vi "transceive.vi"() -> ()   [LabVIEW 2020]
uses:
  <vilib>/measure/matone.llb/Extract Single Tone Information 1 Chan (CDB).vi
  <vilib>/measure/maspectr.llb/FFT Power Spectrum and PSD for 1 Chan (CDB).vi
  <vilib>/measure/NI_MABase.lvlib
  <vilib>/measure/NI_MAPro.lvlib
panel:
  in  "stop":bool
  out "Package Directory":path
  out "Transmit Stop?":bool
  out "Terminal Output":string
  in  "FMC Parameters":T1={"IP"="169.254.92.202", "Port"=22, "Username"="analog", "Password"="analog", "Tx rfPort"="A", "Tx Frequency"=2400, "Sample Rate"=30.72, "Tx Bandwidth"=18, "Tx Attenuation"=0, "Cyclic?"=TRUE, "Rx rfPort"="A", "Rx Frequency"=2400, "Rx Bandwidth"=18, "Num of Samples"=16384, "RxA Att"=0.0, "Rx Gain"=0.0}
  in  "?":enum32{"Transmitted Data", "Rx Time", "Rx Freq"}(tab)
  out "Transmitted Waveform":waveform(dbl)[](graph)
  out "Received Waveform":dbl[][](graph)
  out "PSD":cluster{"f0":dbl, "df":dbl, "magnitude":dbl[]}(graph)={"f0"=-0.5, "df"=0.0009765625, "magnitude"=[-2.1664662387993214, -11.03031844193236, -16.21298370209194, -4.2080616825271475, -1.8741588804049676, 1.1653000889131602, -1.8891898884953007, -2.864952815094211, -21.184075663903045, -6.459011634389907, -9.425575045654224, -3.690679662683627, -1.9755112973017053, -12.88760998423885, -7.142795197511936, -5.749654993033601, -4.232121719401448, -6.5853324526702135, -16.72201576955071, -9.904618860083986, -3.7536909694395684, -11.12706914338175, -2.8284209492202423, -4.69775383894684, -1.81721905978906, 2.6751922066707197, -6.228922467094204, -8.725900475207114, -3.2266453224266387, 0.7951367070723341, 3.18791480156189, 1.146568401648937, -15.284613684557055, -7.029959998724905, -9.547309724544128, -9.641529484569087, -4.012009186143547, -2.007072588608481, -2.7914766687377783, -2.6237078006362573, -4.309788836088561, -18.475581742500292, -4.870258369106881, -2.025766794368759, -4.321152799180626, -7.919073671305048, -9.634049825771205, -9.066188593143584, -0.5305564612559043, -0.31734285019072245, -2.899678030076754, -4.930580506434592, -5.89966356805042, -7.472329086898343, -3.2393794433644625, 2.8054749156287695, 1.101964532151964, -4.615302488116255, -6.950562817482371, -6.012731538910917, -6.136893822759926, -4.6471679348476655, -1.2244038951072234, -4.415810566038147, -10.277196994849163, -6.747298439500046, -9.345274520940713, -24.63822602993131, -9.626589129035054, -12.030032194659979, -8.307672166916715, -4.925425049785537, -6.599824942748922, -14.48643716405336, -4.097115992439623, -4.577980789198419, -7.890347310753404, -19.88220101638118, -4.378072425832935, -5.46719551585171, -5.179404332980243, -1.0377130577596902, -10.067538970313956, -3.9345824246573313, -7.348762210999691, -4.4813140018042255, -13.322269126358782, -18.614476297439715, -11.901757888638036, -15.494707432373744, -2.5504818043536654, -0.39477467835974145, -2.304623583891613, -1.7011053039774162, -1.0588041474234957, -5.7947060018517025, -6.930737241367428, -11.138280621615529, -3.142790539526048, -4.1349241709963085, -6.493611114179859, -13.668598830892726, -6.06473945193608, -4.573451548903187, -12.681769905622991, -10.520049431046665, -11.196572091425558, -3.080583619040455, -1.1668660568295595, -10.149043360414288, -14.050701122230615, -23.29131249709334, -25.61066622144638, -7.28124149909767, -4.729883842869232, -5.731993156566849, -9.19277681711874, -16.35268142406711, -18.644837970125387, -9.055595050639003, -5.065337383658032, -5.737763649573261, -8.955349256338103, -8.614404932103014, -18.012974581333005, -10.62396244470849, -13.554883384566025, -11.053708375035576, -13.814110268725772, -10.341204454518444, -11.601018866430993, -9.480774966741487, -14.773641827392439, -11.639321854216638, -5.276785459852072, -3.389349753355969, -9.62066285902237, -13.704466876991075, -15.356678941850866, -11.090197312926346, -15.765625988870731, -19.504916189187135, -11.722808010214179, -7.598506986517483, -4.505296743673027, -5.822883424781482, -16.09011596093657, -14.043949050340707, -16.089051948303435, -9.487296265628675, -15.128223317596767, -10.018626031429827, -9.267900156035067, -8.380021959177236, -13.476338432933685, -7.208337471083226, -13.354661158796306, -9.04978003921784, -16.012521467074837, -11.961586037421164, -10.924513690003696, -15.265653652735791, -21.78119293221372, -23.444167957273756, -18.99901373597104, -9.661919978212918, -8.769352364462925, -9.287529637864772, -11.285381835174613, -11.978298753836219, -14.12055103294531, -19.629285771576967, -14.884787585567448, -20.815518177082293, -14.164324358055287, -8.780900988880223, -11.738326415102133, -16.152955231194802, -17.32671574436486, -14.838120659422156, -19.05492324460187, -20.95423425206988, -17.5564628136197, -11.578639978063084, -14.486427948155738, -26.34134938136794, -13.688104874335611, -8.57434558212727, -10.449000554689265, -15.905851233765231, -27.66525811513363, -16.0113299515765, -20.040788269819906, -14.555987823168017, -9.646150758194366, -11.27934438013196, -14.566967642712562, -15.132750471219198, -21.40247412832394, -18.07051340158898, -25.17678076571924, -18.78255043567815, -16.45857022203186, -17.443314784160325, -22.145987897198967, -25.718710724338898, -24.544041374309064, -25.384442312132464, -55.16060392584162, -22.108378284322097, -17.760182487108363, -16.197006612175016, -15.734079533899587, -20.285641706516017, -20.491143754075583, -14.564418592526122, -15.741471379702684, -18.511482132849927, -17.809104927296914, -15.124735483684024, -17.619988546039153, -17.85107813457279, -16.929723198620195, -20.948588507870348, -24.0715805700717, -18.118791892009778, -14.262411465607217, -12.299255622076606, -17.79348030858842, -27.607132100714807, -31.523131614059388, -20.31173109515901, -18.375492924569116, -29.91411408852937, -21.431199855002262, -35.5719476973811, -31.028910314184294, -17.602948806381388, -11.422758376296168, -15.796797787853741, -25.905898919356236, -23.309551487188443, -23.56295813940394, -24.9018395326393, -14.308676256089425, -12.644084832963776, -13.954709280494242, -11.568644948187757, -14.614471395213165, -16.83755663945805, -19.316516942378257, -17.622380146368744, -25.38633973795314, -21.367209508959995, -16.67367263138378, -19.022940164088457, -23.968867457596076, -18.111523749501185, -20.158096530028146, -37.615159078310356, -29.73443523402027, -21.712570154675362, -17.774184712470547, -15.506439974547515, -18.562298886616663, -22.88136665916835, -30.92169802339641, -21.059024146049175, -25.552942745021774, -21.776350752149266, -17.530732077159755, -31.369212824553937, -25.105693408622894, -24.372264823560283, -33.91496361346293, -44.72514042785862, -31.04986529591511, -21.39757719194284, -19.991438630226362, -26.34113093177384, -25.84372064517313, -41.748828296403246, -50.48308638460183, -25.421782746303705, -21.935572022862427, -25.368831172623732, -23.90029815548064, -27.074842703290795, -26.158836731751116, -45.411822297777576, -33.86289987595039, -27.872429800965705, -22.446348719121257, -20.502898835792827, -22.345505115510175, -26.643199128152837, -27.716256183557814, -30.43562805608401, -31.91587304586699, -31.2189770891335, -22.8004431029588, -20.463273944792533, -19.37577279279427, -23.775090890229187, -25.782381831922923, -19.676979008748468, -16.937682367459466, -17.5363763173867, -16.420024272236063, -25.164465188456727, -33.73845657221404, -20.065432217663293, -17.520338123580647, -18.750970185274095, -23.902417125492512, -17.07842144571978, -20.652237374407857, -18.34940376696168, -16.46552380797614, -20.25463508958933, -26.79551422437222, -35.67225613415172, -31.047698747465926, -21.268584472975057, -20.646197880367275, -23.518125515414525, -21.652181944937094, -23.208992746835015, -37.70332329061807, -28.49033175719009, -28.225438942675968, -38.79368719898007, -32.82324235723701, -24.214741268728226, -20.138091046784115, -24.47583216925584, -24.65584570012096, -21.53710617559499, -17.789621621098938, -23.016655485388668, -21.33131937730605, -18.96241963232589, -23.306139096559974, -31.77524183835225, -24.193632784059048, -40.79923068575879, -26.673785570437524, -19.91419651268278, -16.38621957158681, -25.037513134504504, -21.441693933714596, -17.271299896472755, -17.966366237189767, -22.947203587037187, -26.841391787104, -25.131401318506317, -17.174143861917088, -19.48010113279951, -15.986811775906064, -16.423921471328864, -21.19474324485939, -24.998695119051902, -22.54368429728293, -34.599609048332674, -26.642769012904175, -48.90868728146549, -26.424252509374067, -23.09570601456403, -21.44586205990473, -22.631979077558935, -22.630462483605292, -18.558161355724486, -21.21070987996529, -24.809823688147283, -28.111643763530555, -19.430787150252662, -18.934036484398895, -24.313645081015203, -24.052224792946827, -21.337203729576096, -26.310760265974885, -22.265681871887644, -18.12636200878271, -27.04230841618223, -26.78834309227041, -24.489069312961078, -18.71467432413909, -18.000186601341582, -21.258402666356005, -20.09803225228808, -20.166171669936954, -21.910662474230264, -27.805008936103718, -30.295775919638544, -20.355530298871475, -20.549721696850245, -19.177016446993573, -26.180585716564796, -31.99990225622599, -20.495928901318834, -19.893554597731963, -18.704938641767647, -16.266614210124846, -17.448229497012967, -21.23963887047376, -18.537721244758988, -22.59856844148533, -26.275140775135817, -23.8173694717668, -23.823056936129458, -24.637271758212908, -25.128701733314553, -20.061986995540472, -23.119809032129123, -28.36903214359627, -18.956044468969168, -18.702942936200742, -21.472616084356083, -19.327919866021922, -17.959722951763457, -18.591527190818006, -16.95060905889876, -19.32712734745809, -20.427199346264523, -31.226680872777273, -19.837382407924874, -22.60017932903269, -17.052777182725478, -20.40946447735477, -22.068669070393724, -20.81515564316504, -19.577957010052938, -20.099322802621508, -29.548811081650825, -26.12769052797335, -21.553209730395206, -19.13107867141223, -24.260238389039458, -27.286618589764757, -33.55279172848271, -21.272869637317534, -19.784506028159107, -26.78020113379997, -21.69964604589776, -24.629693542604922, -24.654456286565768, -15.229511185702185, -16.569856591164672, -25.727420831633523, -18.439246797446323, -15.41270238647343, -17.64852983558219, -27.525394034322925, -25.86016491040037, -17.034285316493328, -17.216011266586317, -17.77965679548461, -20.652685555422117, -25.11634227732326, -16.27916658908456, -19.904867479703867, -26.431609635922726, -25.400319119572327, -23.56382312081276, -21.874088081526608, -20.444656159001873, -36.40291084543626, -24.113336954401966, -24.9090995163475, -26.811296324942685, -18.85628812055225, -19.92832140194353, -17.719053554863546, -14.28207004215883, -17.01207225133356, -21.95767571091194, -16.83321472682335, -21.318257655642107, -21.987004143790692, -20.85570518163312, -22.09894380747681, -32.55333332110235, -29.72934345817011, -19.516577957830926, -17.287725402033377, -19.426934321453327, -21.876145018073018, -19.838378404678384, -21.294753350895476, -19.61650661591934, -23.735219067619013, -29.79064998014501, -30.65154385931423, -27.296316587055323, -22.463811070536956, -30.029030950678003, -23.723839332019715, -22.619765169322648, -21.87602943201536, -23.979099873473245, -26.33209423472927, -25.28676545037344, -24.513447334225354, -22.613416380850417, -28.445775896897572, -25.371972493999166, -26.95410699887337, -20.15755356935991, -29.342659520737925, -23.117020242869415, -22.600770165956984, -16.453300326319948, -12.132638160056581, -17.688216798310844, -20.33929698675172, -21.29991624897785, -22.229537539795302, -19.096565490704737, -28.140881490251157, -24.5329200204889, -24.27097199644253, -25.230287338715787, -23.43131783256496, -23.685264582837465, -25.877652372642412, -21.466251609993957, -19.76707428321712, -20.327234067749636, -23.16049957461841, -35.334331646673085, -26.20291010968397, -22.48453488096971, -22.521502075182678, -31.36991218027869, -29.541918177609592, -27.017269566287077, -24.165269959775163, -23.285450551161823, -31.1267069312302, -30.101399414709064, -21.41837897037453, -24.58127894254097, -33.675712305331146, -21.683603250949346, -23.46814135803816, -22.272480268297727, -20.303160142138484, -14.79328097819032, -17.54276386963902, -27.578074364075917, -27.188085587652218, -40.81262516669441, -27.1459170953992, -21.75914061223462, -18.91717204529973, -18.273575702330835, -22.64422421590675, -33.87762446569896, -22.226379927385153, -26.73584670700638, -24.67387294131232, -22.4854748232693, -36.31842033155398, -30.32832906473766, -27.623873893988407, -23.706361800320103, -39.28294513403284, -25.16384481375086, -29.14490096855095, -27.276793474720826, -30.22387754994218, -33.745621995360914, -21.13080065751321, -24.57667162525871, -21.40716783191923, -18.853149245032274, -20.87286216504811, -21.089605536097324, -21.433298698688983, -20.017338437952464, -22.091483642076778, -25.528526333253232, -20.9065418192947, -22.109035778048014, -40.61595229692652, -28.819683321057216, -28.16363103438912, -24.279230626850943, -18.06309619127601, -17.410855486281854, -29.253796833041918, -15.404729999237691, -25.143861834805232, -21.028188951021782, -23.59218835305257, -21.578422888284152, -25.68972331648026, -26.019146275513222, -18.029172276285372, -18.48357007669874, -17.659913594769137, -48.2437854268398, -18.302838627462748, -17.299244558802382, -18.627231694186637, -28.351797601823048, -21.655347673997255, -20.591819326458985, -29.42489293970261, -23.852565866915917, -36.15777214928648, -22.207740016509767, -20.296014432154223, -20.246050654007814, -26.856018528183263, -21.86136938534775, -19.244680908410075, -21.51739303579617, -20.056241624973538, -16.7222646629974, -18.859442838455404, -25.83383908787424, -23.305221121213794, -21.304054835291485, -25.820493558938878, -28.414975784284184, -27.767917030563783, -25.11334885337878, -22.792698450445776, -18.87117543186417, -20.73147740979615, -32.045486371077104, -25.098310761925866, -31.20757636259459, -21.387330527574377, -16.321479923262135, -16.58896228553176, -21.980872690771683, -42.02788785685936, -30.0006515278838, -18.757620854775755, -16.132462274618096, -23.637414124897695, -27.090364473222294, -21.86531457900997, -17.77321919544772, -16.949862714570273, -15.238539467356684, -15.730773682368644, -16.268405755729283, -17.328384424079417, -21.12891909300498, -20.194319845541898, -22.990301321132684, -27.632872106625342, -29.815486020850347, -53.437609513552296, -25.099883348901106, -28.050249905227513, -25.238353941682053, -18.920387452326143, -17.793562875056107, -18.05827559162568, -17.892584293097112, -23.626797056568552, -21.068850797989004, -19.37995435619343, -17.968181539408256, -15.534487272520627, -17.859497797480593, -22.742065600500155, -29.68362094699843, -24.635890295626982, -24.95482198228014, -24.38034414388111, -23.142504921877823, -18.86511676205624, -20.714811588589768, -24.28716238162186, -22.581457510652733, -28.731877346888396, -19.648954736106063, -24.61884036783917, -27.656612668890475, -19.40140716472233, -19.014493078107378, -29.674178521738995, -21.8969155384475, -19.99872387050329, -20.113178624244163, -21.9286770705693, -22.17623857618413, -24.910673474305725, -32.006128676967755, -23.41505068127347, -23.712189683586185, -29.899969415091476, -27.48158039751953, -27.706718959196195, -22.660148705331295, -19.40529056820971, -24.003963358719954, -28.86174279270587, -25.39456144991061, -28.023212416632308, -27.397584321546702, -28.638365635705302, -26.701711021434992, -37.32014723158207, -32.91599593470649, -33.21925099937459, -31.30991033598654, -31.2280941526455, -20.433366479115286, -19.87291267817699, -21.420416021206407, -17.33516761884006, -22.71233508900824, -24.419666766742655, -24.497763077045576, -24.5490781764792, -26.39950198033429, -24.715884025792644, -23.470016378188568, -21.382443036760783, -22.079530067255796, -18.561108520016898, -25.229058260292426, -24.802846865135237, -27.747385291793186, -27.20581202830468, -27.037703106072904, -19.47500379320967, -24.933467097925423, -21.915665157071697, -27.722597667704694, -20.20533713851103, -18.335532254847557, -20.205255402457034, -29.50280452603961, -25.68574081682002, -15.534415835980404, -13.405087901322457, -17.966232093133865, -26.798692490445877, -21.361673217922288, -15.429928071785666, -16.617493060665776, -27.080951843330816, -35.55964480499562, -26.547786417485064, -30.874533847630143, -23.306145626477832, -21.528398012495234, -31.90664483731751, -39.413438510354595, -19.3194963884024, -25.98808765766458, -26.606742660761906, -20.153792841684147, -19.613736231150096, -18.250265059418325, -27.097889502508735, -25.457471054870595, -28.02615784823974, -20.712914859368574, -23.062885911033568, -27.647652753943493, -21.757064606943942, -20.515510787449482, -21.148972569068505, -17.163549389658655, -14.128322318033199, -14.708517110823587, -21.13233507351331, -20.99462533980155, -11.033770144491386, -9.51961262575132, -19.740675685913384, -21.15896715801221, -18.272470374521454, -33.23019811130402, -20.817362450813217, -30.02135754202454, -19.3676160404167, -18.933303658417763, -21.889997993019634, -25.79689099190281, -25.65701279491698, -20.447890468062575, -17.507290471317308, -13.016197741038438, -11.67217989493539, -20.96905894781075, -15.26695904037564, -11.4928076833581, -12.775856238826167, -19.148804977158974, -26.141184946414917, -14.794321978537665, -14.630894652485583, -18.851782382867228, -35.95721775968208, -21.852054071099722, -35.02840377017914, -33.64524346727479, -16.667045609645605, -12.876582667152851, -27.10253350692326, -13.519096734706933, -13.705405718252635, -24.963565579903538, -19.683851297291618, -12.205992795378918, -18.59934714029558, -12.578055400486878, -11.504072751432535, -14.402436233715882, -14.72501828474037, -16.63278860038672, -18.861702859403117, -25.88686529313735, -19.907219992058177, -15.568133442373313, -23.923011018364004, -14.176535562048283, -20.10657406962344, -10.357388030626016, -12.657468992497659, -19.880786782159593, -36.51382658833635, -18.298507167667122, -23.27195817682455, -20.195750507226414, -26.439125545441197, -23.263807420996518, -19.71905947565326, -20.270513733655786, -26.57460056122364, -21.03782364768375, -14.256647108137877, -9.696558647379668, -11.959207929169173, -19.152133333871856, -8.36216215521305, -9.116402131835802, -26.211214225343156, -25.831788615717123, -19.342433244022786, -17.164435757532274, -8.518057904863127, -8.471255034930937, -10.9175696443224, -16.075978391408892, -15.94303448996656, -14.661556992979673, -12.019598897788487, -17.485937277881135, -20.190327838373797, -9.233558136182532, -11.826521061283925, -16.392083871014325, -12.987000436100525, -6.697949642770569, -6.58684419944123, -24.58333891872226, -10.312611361513026, -13.72815212792301, -5.0062459888898045, -5.064071908964473, -7.794898929398192, -9.356565144273999, -15.082162785986293, -20.57522382578895, -18.55422200515601, -20.43260644178257, -35.31186779146302, -14.99246336464994, -15.133079689334046, -14.837346810136136, -5.946269161431409, -8.635805512458468, -15.270250938725225, -10.562523393130373, -16.435574314475325, -13.864613372382859, -5.050816029531173, -3.8535079147378797, -6.971313195865286, -10.505597319470418, -7.716526685849176, -11.31165398880966, -11.294717090933041, -6.112285229509934, -7.254046050138914, -15.857165395849407, -9.60448244993986, -7.180320192968283, -6.843234544165839, -11.248952703933597, -16.3443500737425, -10.732735820207758, -22.74869768064631, -22.45531897544403, -8.80636080387957, -14.038961829474232, -10.662098986203096, -9.448711745336523, -13.485143627949645, -28.21500937388383, -18.20928095094015, -7.983685730367764, -3.9272167962407285, -13.735674790679296, -10.630605969311222, -10.555498965455444, -4.6272482134731625, -4.083587423538876, -14.612923671431112, -14.018697867250488, -9.726951043776781, -2.0210656192074747, -2.1009573356943942, -9.261798408117622, -7.209873050924771, -16.76975868585653, -3.6435929736898327, -2.7054047125736918, -18.281248142217283, -8.548746264061602, -24.31838624093668, -20.71372555847999, -8.489300198316576, -10.135789453673986, -10.223545857784393, -14.412075018459573, -11.358057392185572, -8.198146753254395, -5.437541113037641, -16.073500085531897, -4.471994279259307, -5.185281044275124, -16.3315910930994, -2.0143348019626086, -1.608326704173825, -10.445059671578012, -11.824051886863796, -5.4390683344730135, -3.356908890334393, -7.43386703544929, -25.09865558366144, -20.017724982762925, -11.359608058485222, -6.6289009205371165, -5.811321297722685, -7.649369982719586, -5.506350366954667, -6.818978299565705, -1.4769809430036227, -9.308719252907155, -4.353949417319006, -0.11501051519774996, -2.2038443609504204, -6.181875808817359, -16.211162929226678, -5.195318273119352, -11.270032894141051, -9.998002263416993, -3.199826431151937, -1.5018070529485803, -9.280780742295493, -23.665408085418, -11.405315221474687, -2.170857177497663, -1.4425459855181268, -4.335590280563005, -2.7837979397506207, -4.401963322808209, -7.952431326868934, -20.89457317234706, -11.269737903670032, -5.842090314145938, -8.273674602539744, -5.064681488690899, -12.86078186182105, -1.3106254458914477, -4.349907246750549, -6.504857181138518, -15.86623631447427, -3.9335952874878286, -0.4735191748974057, -3.090263685516819, -4.2417198265679605, -11.908089563935638, -12.668945570630243, -17.033791589100527, -7.09341804926007, 0.16676594388460936, -0.8886131593434281, -0.6473106312266131, -0.573142409427389, -8.708059058862286, -10.261293939709237, -1.1366006946455052, 4.143416046858032, 4.0031594116978155, -2.992142727926834, -10.541787110026132, -5.224092817584797, -9.321263827756663, -3.7195918719691674, -0.3528685692882417, -14.013593255320185, -8.735632191402567, -11.804551821115794, -2.8134392445446235, -4.486861584527423, -6.354994609223246, -11.280313560560359, -2.24150871938288, -14.781061946184895, -6.378925464861641, -39.628361231840756, 1.623285802436084]}
  out "Peak Frequency":dbl format="%.2p"
  out "Error Out":errorcluster
  # "Tx Config"
  # "Rx Config"
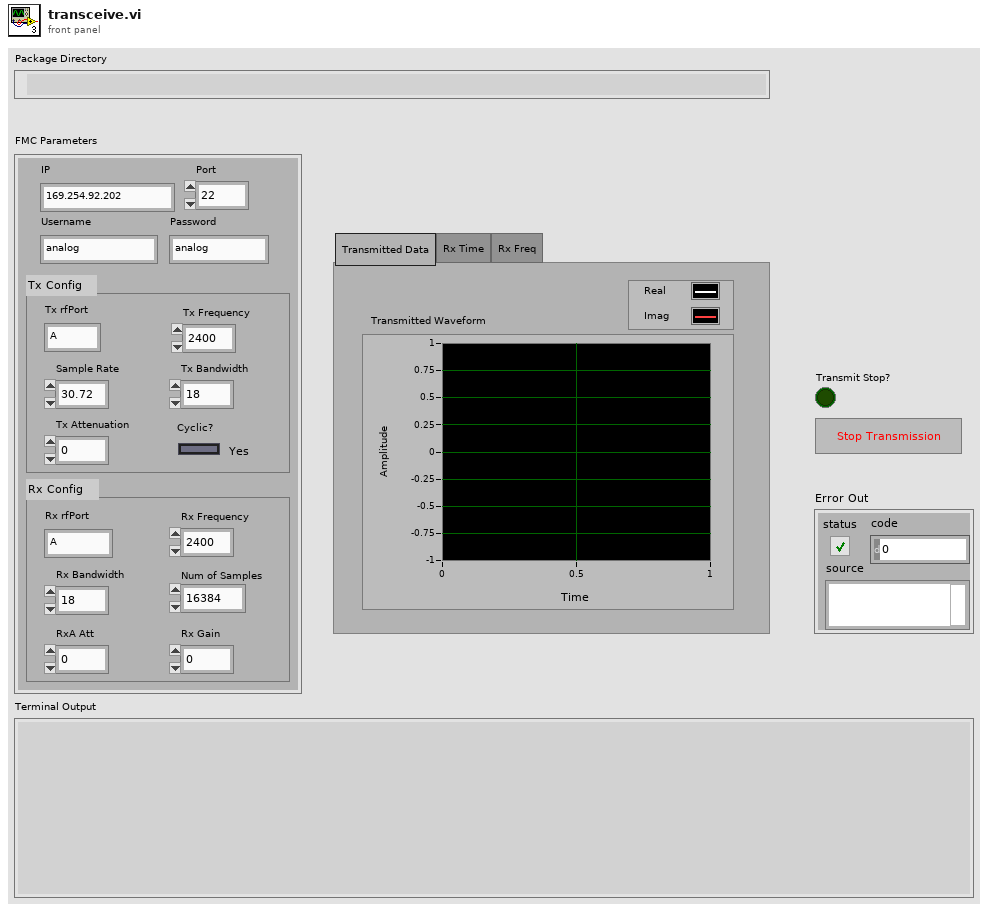
[diagram p1: front panel]
types:
  T1 = cluster{"IP":string, "Port":i32, "Username":string, "Password":string, "Tx rfPort":string, "Tx Frequency":i64, "Sample Rate":dbl, "Tx Bandwidth":i32, "Tx Attenuation":i32, "Cyclic?":bool, "Rx rfPort":string, "Rx Frequency":i64, "Rx Bandwidth":i32, "Num of Samples":i64, "RxA Att":dbl, "Rx Gain":dbl}
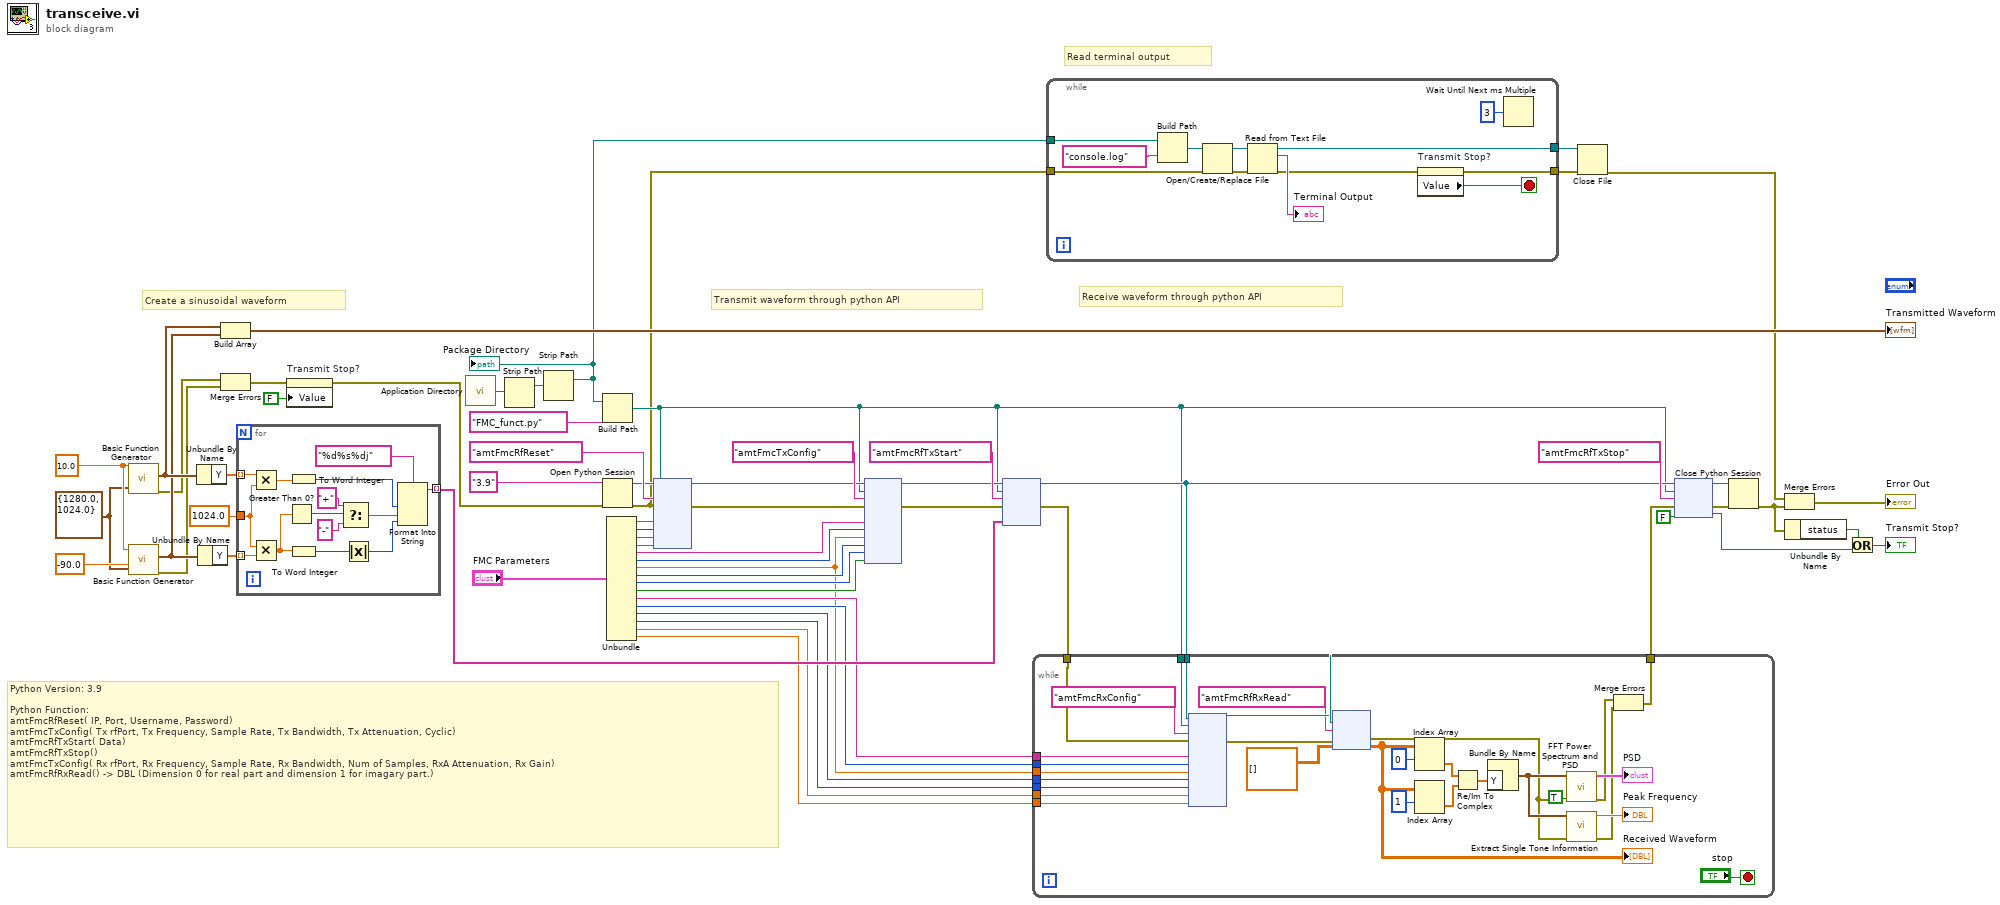
[diagram p0: block diagram]
diagram:
  w62 = 10.0 ("frequency")
  w60 = cluster{"Fs":dbl, "#s":dbl} {"Fs"=1280.0, "#s"=1024.0} ("sampling info")
  # "Read terminal output"
  # "Python Version: 3.9\n\nPython Function:\namtFmcRfReset( IP, Port, Username, Password)\namtFmcTxConfig( Tx rfPort, Tx Frequency, Sample Rate, Tx Bandwidth, Tx Attenuation, Cyclic)\namtFmcRfTxStart( Data)\namtFmcRfTxStop()\namtFmcTxConfig( Rx rfPort, Rx Frequency, Sample Rate, Rx Bandwidth, Num of Samples, RxA Attenuation, Rx Gain)\namtFmcRfRxRead() -> DBL (Dimension 0 for real part and dimension 1 for imagary part.)"
  # "Receive waveform through python API"
  # "Transmit waveform through python API"
  # "Create a sinusoidal waveform"
  n1 = call <vilib>:"Basic Function Generator.vi"("sampling info"=w60, "frequency"=w62) -> ("error out"=w4:errorcluster, "signal out"=w56:waveform(dbl))  [unwired: 7 in, 1 out]
  n2 = call <vilib>:"Basic Function Generator.vi"("sampling info"=w60, "phase"=-90.0, "frequency"=w62) -> ("error out"=w3:errorcluster, "signal out"=w55:waveform(dbl))  [unwired: 6 in, 1 out]
  n3 = Unbundle By Name(w56) -> ("Y"=w58:dbl[])
  n4 = Unbundle By Name(w55) -> ("Y"=w57:dbl[])
  n5 = Build Array(w56, w55) -> (→"Transmitted Waveform":waveform(dbl)[])
  n6 = Merge Errors(w4, w3) -> (w2:errorcluster)
  n7 = for {
    tunnel: w57 -> [w76] mode=indexing
    tunnel: w58 -> [w75] mode=indexing
    tunnel: 1024.0 -> [w74]
    tunnel: [w65] -> w32 mode=indexing
    n8 = Multiply(x=w75, y=w74) -> (x*y=w72:dbl)
    n9 = Multiply(x=w74, y=w76) -> (x*y=w71:dbl)
    n10 = Greater Than 0?(x=w71) -> (x > 0?=w73:bool)
    n11 = To Word Integer(number=w72) -> (16bit integer=w69:i16)
    n12 = To Word Integer(number=w71) -> (16bit integer=w63:i16)
    n13 = Select(t="+", s=w73, f="-") -> (s? t:f=w70:string)
    n14 = Absolute Value(x=w63) -> (abs(x)=w64:i16)
    n15 = Format Into String(format string="%d%s%dj", w69, w70, w64) -> (resulting string=w65:string)  [unwired: 2 in, 1 out]
  }
  n16 = property on="Transmit Stop?" class="Bool (strict)"(error in=w2, "Value"=FALSE) -> (error out=w1:errorcluster)  [unwired: 1 in, 1 out]
  n17 = call <vilib>:"Application Directory.vi"() -> ("Application Directory"=w14:path)
  n18 = Strip Path(path=w14) -> (stripped path=w13:path)  [unwired: 1 out]
  n19 = Strip Path(path=w13) -> (stripped path=w12:path)  [unwired: 1 out]
  "Package Directory" <- w12
  n20 = Build Path(base path=w12, name or relative path="FMC_funct.py") -> (appended path=w22:path)
  n21 = Open Python Session(python version="3.9" ("Python version"), 3:w1) -> (session out=w33:refnum<k35>, error out=w15:errorcluster)  [unwired: 1 in]
  n22 = Unbundle("FMC Parameters") -> ("IP"=w45:string, "Port"=w46:i32, "Username"=w47:string, "Password"=w48:string, "Tx rfPort"=w49:string, "Tx Frequency"=w50:i64, "Sample Rate"=w27:dbl, "Tx Bandwidth"=w51:i32, "Tx Attenuation"=w52:i32, "Cyclic?"=w53:bool, "Rx rfPort"=w29:string, "Rx Frequency"=w28:i64, "Rx Bandwidth"=w26:i32, "Num of Samples"=w25:i64, "RxA Att"=w24:dbl, "Rx Gain"=w23:dbl)
  n23 = node(w33, w22, "amtFmcRfReset" ("function name"), w15, w45, w46, w47, w48) -> (w38:refnum<k35>, w43:errorcluster)  [unwired: 6 in, 2 out]
  n24 = node(w38, w22, "amtFmcTxConfig" ("function name"), w43, w49, w50, w27, w51, w52, w53) -> (w39:refnum<k35>, w44:errorcluster)  [unwired: 8 in, 2 out]
  n25 = node(w39, w22, "amtFmcRfTxStart" ("function name"), w44, w32) -> (w30:refnum<k35>, w31:errorcluster)  [unwired: 3 in, 2 out]
  n26 = while {
    tunnel: w31 -> [w106]
    tunnel: w30 -> [w105]
    tunnel: w29 -> [w104]
    tunnel: w28 -> [w103]
    tunnel: w27 -> [w102]
    tunnel: w26 -> [w101]
    tunnel: w25 -> [w100]
    tunnel: w24 -> [w99]
    tunnel: w23 -> [w98]
    tunnel: w22 -> [w97]
    tunnel: [w96] -> w7
    stop <- "stop" stop-if-true
    n27 = node(w105, w97, "amtFmcRxConfig" ("function name"), w106, w104, w103, w102, w101, w100, w99, w98) -> (w95:refnum<k35>, w94:errorcluster)  [unwired: 9 in, 2 out]
    n28 = node(w95, w97, "amtFmcRfRxRead" ("function name"), w94, dbl[][] []) -> (w80:errorcluster, w81:dbl[][])  [unwired: 3 out]
    "Received Waveform" <- w81
    n29 = Index Array(array=w81, index (row)=0) -> (element=w86:dbl[])  [unwired: 1 in]
    n30 = Index Array(array=w81, index (row)=1) -> (element=w85:dbl[])  [unwired: 1 in]
    n31 = Re/Im To Complex(1:w85, 2:w86) -> (0:w91:cdb[])
    n32 = Bundle By Name("Y"=w91) -> (w90:waveform(cdb))  [unwired: 1 in]
    n33 = call-poly <vilib>:"FFT Power Spectrum and PSD.vi"("error in (no error)"=w80, "dB On (F)"=TRUE, "time signal"=w90) -> ("error out"=w78:errorcluster, "Power Spectrum / PSD"=→"PSD":cluster{"f0":dbl, "df":dbl, "magnitude":dbl[]})  [unwired: 5 in, 2 out]
    n34 = call-poly <vilib>:"Extract Single Tone Information.vi"("error in (no error)"=w80, "time signal in"=w90) -> ("error out"=w79:errorcluster, "detected frequency"=→"Peak Frequency":dbl)  [unwired: 4 in, 4 out]
    n35 = Merge Errors(w78, w79) -> (w96:errorcluster)
  }
  n36 = while {
    tunnel: [w109] -> w18
    tunnel: [w114] -> w17
    tunnel: w12 -> [w112]
    tunnel: w15 -> [w107]
    stop <- w108 stop-if-true
    n37 = Build Path(base path=w112, name or relative path="console.log" ("function name")) -> (appended path=w117:path)
    n38 = Open/Create/Replace File(file path (use dialog)=w117, error in=w107) -> (refnum out=w113:refnum<file>, error out=w115:errorcluster)  [unwired: 4 in, 1 out]
    n39 = Read from Text File(file (use dialog)=w113, error in=w115) -> (refnum out=w114:refnum<file>, text=→"Terminal Output":string, error out=w110:errorcluster)  [unwired: 2 in, 1 out]
    n40 = property on="Transmit Stop?" class="Bool (strict)"(error in=w110) -> (error out=w109:errorcluster, "Value"=w108:bool)  [unwired: 1 in, 1 out]
    n41 = Wait Until Next ms Multiple(millisecond multiple=u32 3) -> ()  [unwired: 1 out]
  }
  n42 = Close File(refnum=w17, error in=w18) -> (error out=w16:errorcluster)  [unwired: 1 out]
  n43 = node(w30, w22, "amtFmcRfTxStop" ("function name"), w7, FALSE ("dB On (F)")) -> (w21:refnum<k35>, w20:errorcluster, w8:bool)  [unwired: 2 out]
  n44 = Close Python Session(session in=w21, error in=w20) -> (11:w6:errorcluster)
  n45 = Merge Errors(w16, w6) -> (→"Error Out":errorcluster)
  n46 = Unbundle By Name(w6) -> ("status"=w9:bool)
  n47 = Or(x=w9, y=w8) -> (x .or. y?=→"Transmit Stop?":bool)
